vi "Case Structure.vi"() -> ()   [LabVIEW 2022 SP3]
panel:
  out "T":dbl(slide) scale=0.0..100.0
  out "T":string
  out "C":string
  in  "F?":dbl
  in  "stop":bool
  in  "C":dbl(slide) scale=0.0..10.0
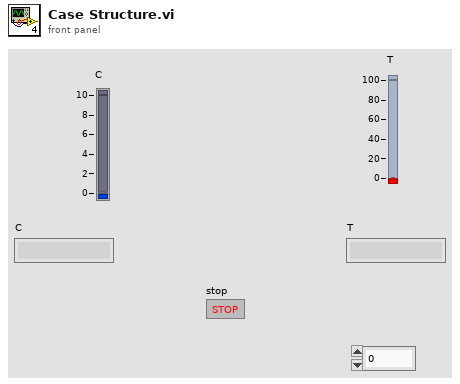
[diagram p1: front panel]
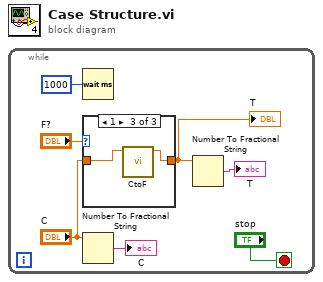
[diagram p0: block diagram]
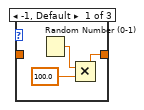
[diagram p2: hidden frame]
diagram:
  n1 = while {
    stop <- "stop" stop-if-true
    n2 = Wait (ms)(milliseconds to wait=u32 1000) -> ()  [unwired: 1 out]
    n3 = case shown="1" "F?" {
      tunnel: "C" -> [_ w11 w12]
      tunnel: [w10 w11 w13] -> w1
      frame -1, Default {
        n4 = Random Number (0-1)() -> (number: 0 to 1=w9:dbl)
        n5 = Multiply(x=w9, y=100.0) -> (x*y=w10:dbl)
      }
      frame 0 {
      }
      frame 1 {
        n6 = call "CtoF.vi"("Celsius"=w12) -> ("Fahrenheit"=w13:dbl)  [unwired: 9 in]
      }
    }
    "T" <- w1
    n7 = Number To Fractional String(number="C") -> (F-format string=→"C":string)  [unwired: 3 in]
    n8 = Number To Fractional String(number=w1) -> (F-format string=→"T":string)  [unwired: 3 in]
  }
